vi "Set Power.vi"(8 "error in (no error)":errorcluster, 9 "Right Power":dbl(slide) min=-1.0 max=1.0 step=0.1 scale=-1.0..1.0, 10 "Left Power":dbl(slide) min=-1.0 max=1.0 step=0.1 scale=-1.0..1.0, 11 "Drive Train in":refnum<class "Drive Train.lvclass">) -> (0 "error out":errorcluster, 3 "Drive Train out":refnum<class "Drive Train.lvclass">)   [LabVIEW 2013, in "Logical Systems.lvlib" / "Drive Train.lvlib" / "Drive Train.lvclass"]
uses:
  Drive Train.lvclass
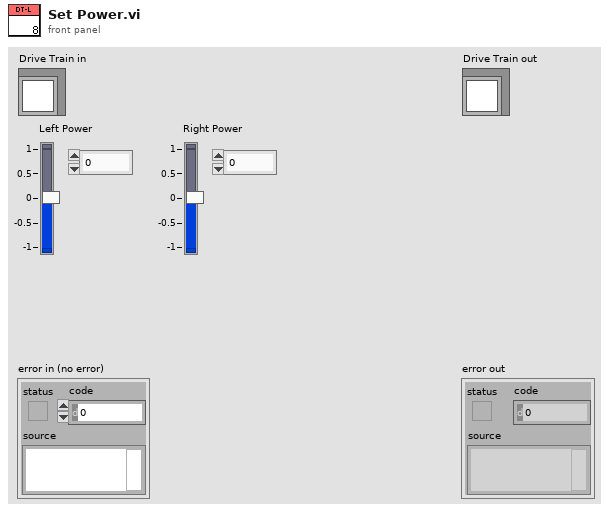
[diagram p1: front panel]
types:
  T1 = typedef "Logical Systems.lvlib/Drive Train.lvlib/Drive Train.lvclass/Drive Train Status.ctl" = cluster{"Left Power":dbl, "Right Power":dbl, "Left Power Setpoint":dbl, "Right Power Setpoint":dbl}
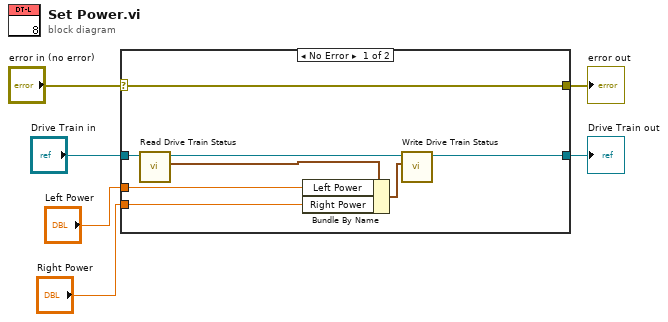
[diagram p0: block diagram]
diagram:
  n1 = case shown="No Error" "error in (no error)" {
    selector: "error in (no error)" -> [w14 w16]
    tunnel: [w14 w16] -> w5
    tunnel: [w11 w15] -> w3
    tunnel: "Drive Train in" -> [w13 w15]
    tunnel: "Left Power" -> [w8 _]
    tunnel: "Right Power" -> [w7 _]
    frame No Error {
      n2 = call-dynamic "Read Drive Train Status.vi"("Drive Train in"=w13) -> ("Drive Train Status"=w10:T1, "Drive Train out"=w12:refnum<class "Drive Train.lvclass">)  [unwired: 8 in, 1 out]
      n3 = Bundle By Name(cluster=w10, "Left Power"=w8, "Right Power"=w7) -> (w9:T1)
      n4 = call-dynamic "Write Drive Train Status.vi"("Drive Train Status"=w9, "Drive Train in"=w12) -> ("Drive Train out"=w11:refnum<class "Drive Train.lvclass">)  [unwired: 8 in, 1 out]
    }
    frame Error {
    }
  }
  "error out" <- w5
  "Drive Train out" <- w3
